vi "KCube Sensor.vi"() -> ()   [LabVIEW 2025]
uses:
  \\chem-fs-prd-01\cyran_research/Users/Erykah F/Vertical Stage + Sensor/Thorlabs.MotionControl.Controls.dll
  Vertical Stage + Sensor/Thorlabs.MotionControl.Controls.dll
  \\chem-fs-prd-01\cyran_research/Users/Erykah F/Vertical Stage + Sensor/ThorLabs.MotionControl.KCube.PositionAlignerCLI.dll
  Vertical Stage + Sensor/ThorLabs.MotionControl.KCube.PositionAlignerCLI.dll
panel:
  out "Demand Y":dbl
  out "Demand X":dbl
  out "Y diff":dbl
  out "X diff":dbl
  out "Sum":dbl
  in  "Exit":bool
  in  "KCube Serial  Number":string="69254064"
  in  "KCubePositionAlignerControl":refnum<k24>(container)
  # "Sum voltage"
  # "These are their differences...?"
  # "Maybe these are their actual positions?"
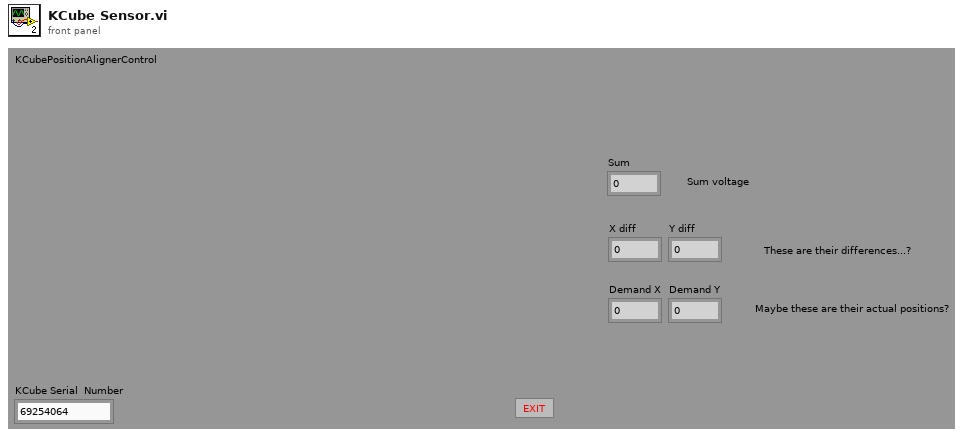
[diagram p1: front panel]
types:
  T1 = cluster{"KCubePositionAlignerControl":refnum<k24>, "Device":refnum<k24>}
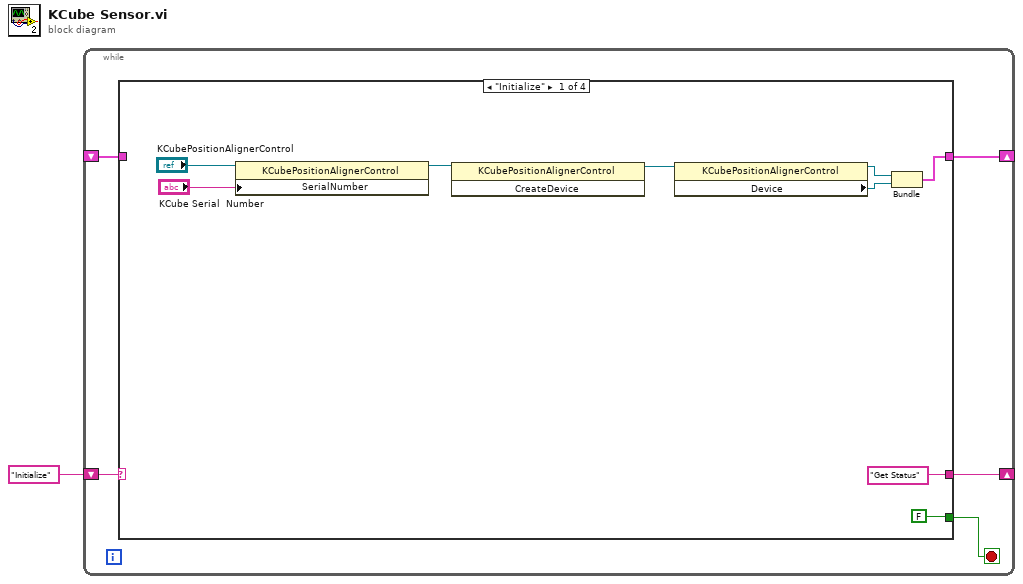
[diagram p0: block diagram]
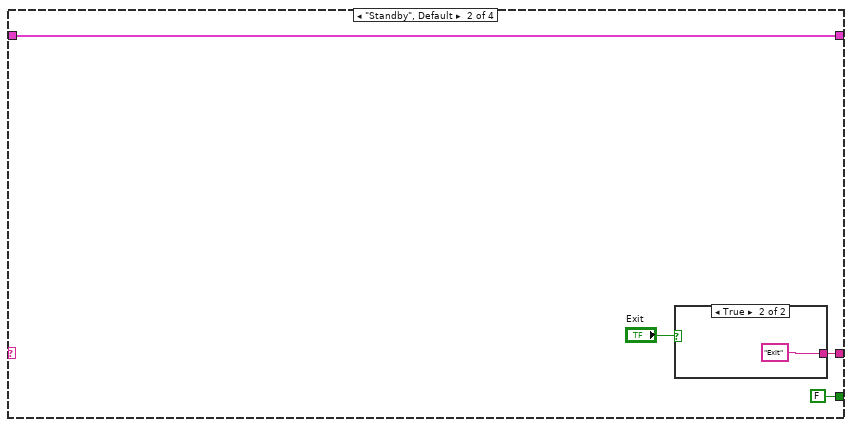
[diagram p2: hidden frame]
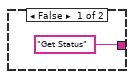
[diagram p3: hidden frame]
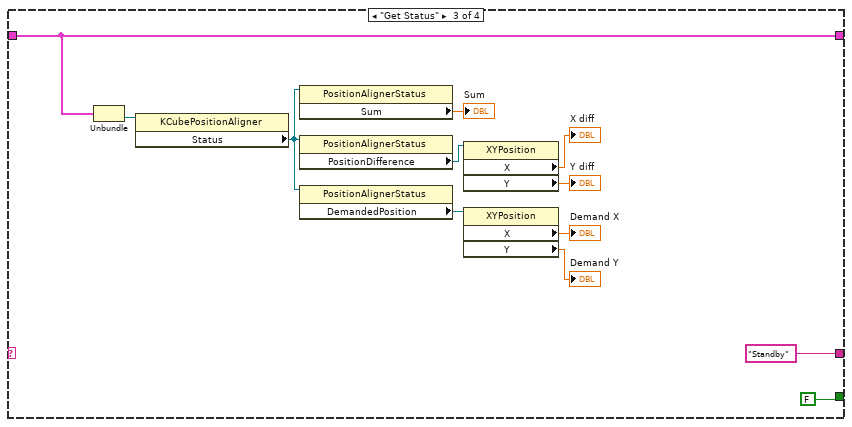
[diagram p4: hidden frame]
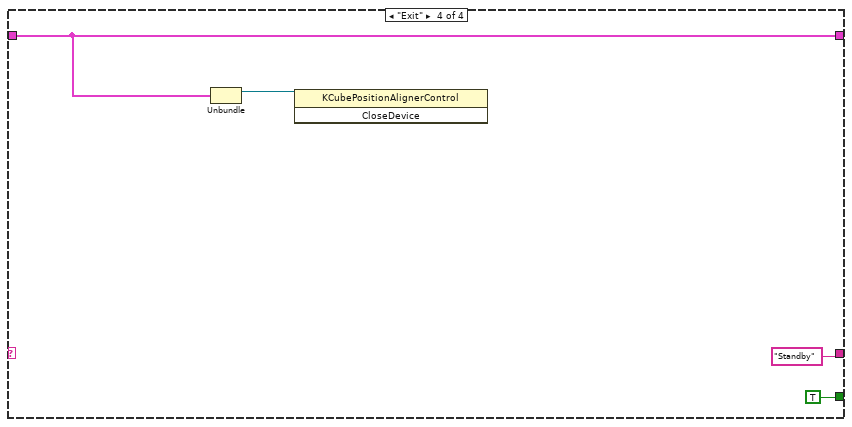
[diagram p5: hidden frame]
diagram:
  n1 = while {
    shift-right: [w5] -> _
    shift-left: "Initialize" -> [w6]
    shift-right: [w3] -> _
    shift-left: _ -> [w2]
    stop <- w4 stop-if-true
    n2 = case shown="\"Initialize\"" w6 {
      tunnel: ["Get Status" w18 "Standby" "Standby"] -> w5
      tunnel: [FALSE FALSE FALSE TRUE] -> w4
      tunnel: [w8 w16 w25 w35] -> w3
      tunnel: w2 -> [_ w16 w25 w35]
      frame "Initialize" {
        n3 = property class="KCubePositionAlignerControl"(reference="KCubePositionAlignerControl", "SerialNumber"="KCube Serial  Number") -> (reference out=w14:refnum<k24>)  [unwired: 1 in, 1 out]
        n4 = invoke class="KCubePositionAlignerControl" method="CreateDevice"(reference=w14) -> (reference out=w13:refnum<k24>)  [unwired: 2 in, 2 out]
        n5 = property class="KCubePositionAlignerControl"(reference=w13) -> (reference out=w10:refnum<k24>, "Device"=w9:refnum<k24>)  [unwired: 1 in, 1 out]
        n6 = Bundle("KCubePositionAlignerControl"=w10, "Device"=w9) -> (w8:T1)  [unwired: 1 in]
      }
      frame "Standby", Default {
        n7 = case shown="True" "Exit" {
          tunnel: ["Get Status" "Exit"] -> w18
          frame False {
          }
          frame True {
          }
        }
      }
      frame "Get Status" {
        n8 = Unbundle(w25) -> ("Device"=w23:refnum<k24>)  [unwired: 1 out]
        n9 = property class="KCubePositionAligner"(reference=w23) -> ("Status"=w22:refnum<k24>)  [unwired: 1 in, 2 out]
        n10 = property class="PositionAlignerStatus"(reference=w22) -> ("Sum"=→"Sum":dbl)  [unwired: 1 in, 2 out]
        n11 = property class="PositionAlignerStatus"(reference=w22) -> ("PositionDifference"=w27:refnum<k24>)  [unwired: 1 in, 2 out]
        n12 = property class="PositionAlignerStatus"(reference=w22) -> ("DemandedPosition"=w26:refnum<k24>)  [unwired: 1 in, 2 out]
        n13 = property class="XYPosition"(reference=w27) -> ("X"=→"X diff":dbl, "Y"=→"Y diff":dbl)  [unwired: 1 in, 2 out]
        n14 = property class="XYPosition"(reference=w26) -> ("X"=→"Demand X":dbl, "Y"=→"Demand Y":dbl)  [unwired: 1 in, 2 out]
      }
      frame "Exit" {
        n15 = Unbundle(w35) -> ("KCubePositionAlignerControl"=w34:refnum<k24>)  [unwired: 1 out]
        n16 = invoke class="KCubePositionAlignerControl" method="CloseDevice"(reference=w34) -> ()  [unwired: 2 in, 3 out]
      }
    }
  }
